vi "ExCircularBufROI.vi"() -> ()   [LabVIEW 2010]
panel:
  in  "X Start":u32=1 min=1 step=1
  in  "Y Bin":u32=1 min=1 step=1
  in  "X End":u32=1 min=1 step=1
  in  "X Bin":u32=1 min=1 step=1
  in  "Y Start":u32=1 min=1 step=1
  in  "Y End":u32=1 min=1 step=1
  in  "Intensifier":bool
  in  "Temperature":dbl=-10.0 format="%.2f"
  in  "Exposure":dbl min=0.0 step=0.001 format="%.3f"
  in  "stop":bool
  in  "Store":bool
  out "error out":errorcluster
  in  "error in (no error)":errorcluster
  # "ExCircularBufROI:\nThis example allows a single ROI\nto be programmed up. It then runs\nin sync (focus) mode displaying \nthe ROI data as it comes in.\nNote: this example requires the \ncamera support circular buffers."
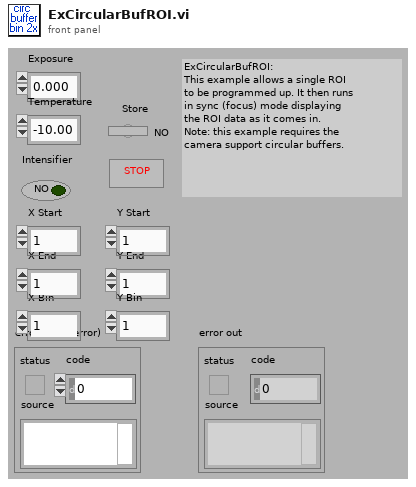
[diagram p1: front panel]
types:
  T1 = cluster{"X Start":u32, "X End":u32, "X Bin":u32, "Y Start":u32, "Y End":u32, "Y Bin":u32}
  T2 = cluster{"acquire focus mode":u32, "Exposure":dbl, "Number of Images":u32, "Software accumulation":u32}
  T3 = cluster{"Camera Handle":u32, "Pulser Handle":u32, "File Handle":u32, "Display Handle":u32, "Image Handle":u32}
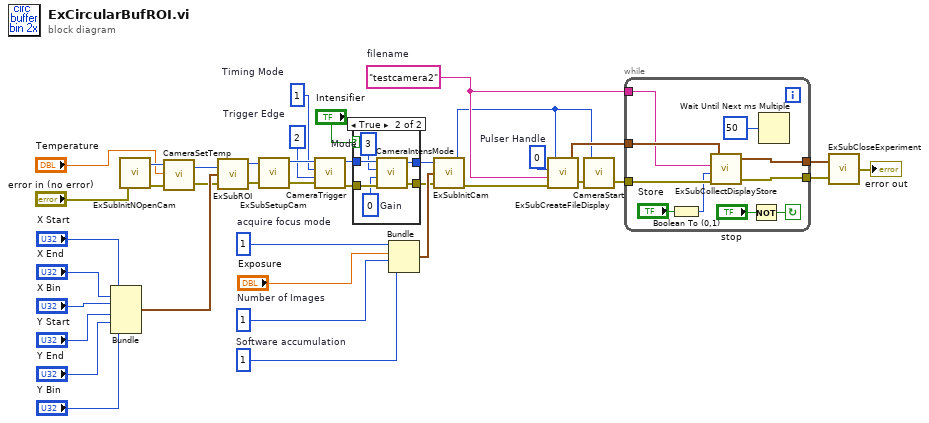
[diagram p0: block diagram]
diagram:
  w22 = u32 0  # Pulser Handle
  w23 = u32 1  # Timing Mode
  w24 = u32 2  # Trigger Edge
  w27 = u32 1  # acquire focus mode
  w26 = u32 1  # Number of Images
  w25 = u32 1  # Software accumulation
  w39 = "testcamera2"  # filename
  n1 = Bundle("X Start"="X Start", "X End"="X End", "X Bin"="X Bin", "Y Start"="Y Start", "Y End"="Y End", "Y Bin"="Y Bin") -> (w9:T1)  [unwired: 1 in]
  n2 = call "ExSubInitNOpenCam.vi"("error in (no error)"="error in (no error)") -> ("Camera Handle"=w6:u32, "error out"=w7:errorcluster)
  n3 = call <userlib>:"CameraSetTemp.vi"("error in (no error)"=w7, "Temperature"="Temperature", "Camera Handle"=w6) -> ("error out"=w5:errorcluster, "Camera Handle"=w4:u32)
  n4 = call "ExSubROI.vi"("error in (no error)"=w5, "ROI"=w9, "Camera Handle"=w4) -> ("error out"=w2:errorcluster, "Camera Handle"=w8:u32)
  n5 = call "ExSubSetupCam.vi"("error in (no error)"=w2, "Camera Handle"=w8) -> ("error out"=w1:errorcluster, "Camera Handle"=w30:u32)
  n6 = call <userlib>:"CameraTrigger.vi"("error in"=w1, "Trigger Edge"=w24, "Timing Mode"=w23, "Camera Handle"=w30) -> ("error out"=w18:errorcluster, "Camera Handle"=w20:u32)
  n7 = case shown="True" "Intensifier" {
    tunnel: w20 -> [w41 w47]
    tunnel: [w41 w46] -> w19
    tunnel: w18 -> [w40 w45]
    tunnel: [w40 w44] -> w17
    frame False {
    }
    frame True {
      w42 = u32 0  # Gain
      w43 = u32 3  # Mode
      n8 = call <userlib>:"CameraIntensMode.vi"("error in"=w45, "Intensifier Gain"=w42, "Mode"=w43, "Camera Handle"=w47) -> ("error out"=w44:errorcluster, "Camera Handle"=w46:u32)
    }
  }
  n9 = Bundle("acquire focus mode"=w27, "Exposure"="Exposure", "Number of Images"=w26, "Software accumulation"=w25) -> (w36:T2)  [unwired: 1 in]
  n10 = call "ExSubInitCam.vi"("error in (no error)"=w17, "Camera Information"=w36, "Camera Handle"=w19) -> ("error out"=w35:errorcluster, "Camera Handle"=w21:u32)
  n11 = call "ExSubCreateFileDisplay.vi"("error in (no error)"=w35, "File and Display Name"=w39, "Pulser Handle"=w22, "Camera Handle"=w21) -> ("error out"=w28:errorcluster, "Handles Out"=w34:T3)
  n12 = call <userlib>:"CameraStart.vi"("error in"=w28, "Camera Handle"=w21) -> ("error out"=w29:errorcluster)  [unwired: 1 out]
  n13 = while {
    tunnel: w34 -> [w56]
    tunnel: w29 -> [w55]
    tunnel: w39 -> [w48]
    tunnel: [w53] -> w32
    tunnel: [w54] -> w33
    stop <- w51 continue-if-true
    n14 = Boolean To (0,1)(Boolean="Store") -> (0, 1=w49:i16)
    n15 = call "ExSubCollectDisplayStore.vi"("error in (no error)"=w55, "Store flag"=w49, "Display Title"=w48, "Handle Cluster"=w56) -> ("error out"=w53:errorcluster, "Handle Cluster Out"=w54:T3)  [unwired: 1 out]
    n16 = Not(x="stop") -> (.not. x?=w51:bool)
    n17 = Wait Until Next ms Multiple(millisecond multiple=u32 50) -> ()  [unwired: 1 out]
  }
  n18 = call "ExSubCloseExperiment.vi"("error in (no error)"=w32, "Handles In"=w33) -> ("error out"=→"error out":errorcluster)
